vi "_Word Example.vi"() -> ()   [LabVIEW 2017]
uses:
  LabVIEW NPOI/xwpfReader/xwpfReader.lvclass/xwpfReader.ctl
  C:/Users/Neo/Desktop/Dev_Tools_BR/LabVIEW_NPOI/lib/NPOI 2.1.1/NPOI.OOXML.dll
  lib/NPOI 2.1.1/NPOI.OOXML.dll
  LabVIEW NPOI/xwpfReader/Get xwpfRef.vi
  LabVIEW NPOI/Document/Document.lvclass
  LabVIEW NPOI/xwpfReader/xwpfReader.lvclass
panel:
  out "Array 2":i32[][][](array[numeric])
  out "Array 3":string[](array[string])
  out "Array":string[](array[string])
  in  "Text":string="Text ajoute."
  in  "File Path":path
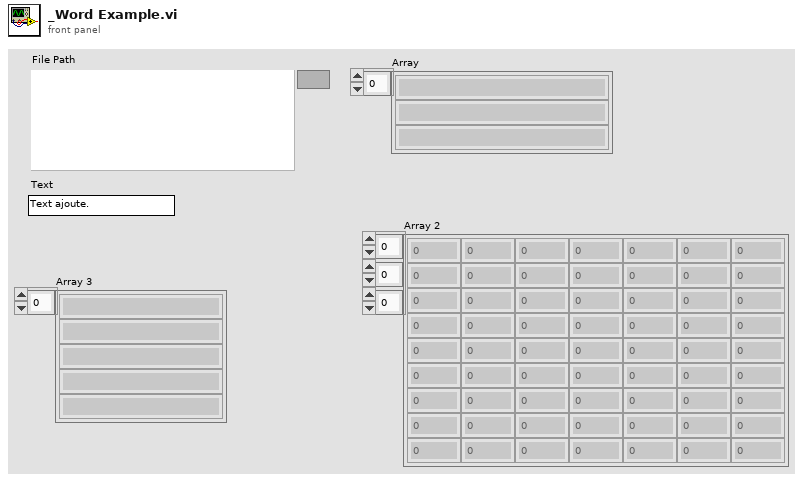
[diagram p1: front panel]
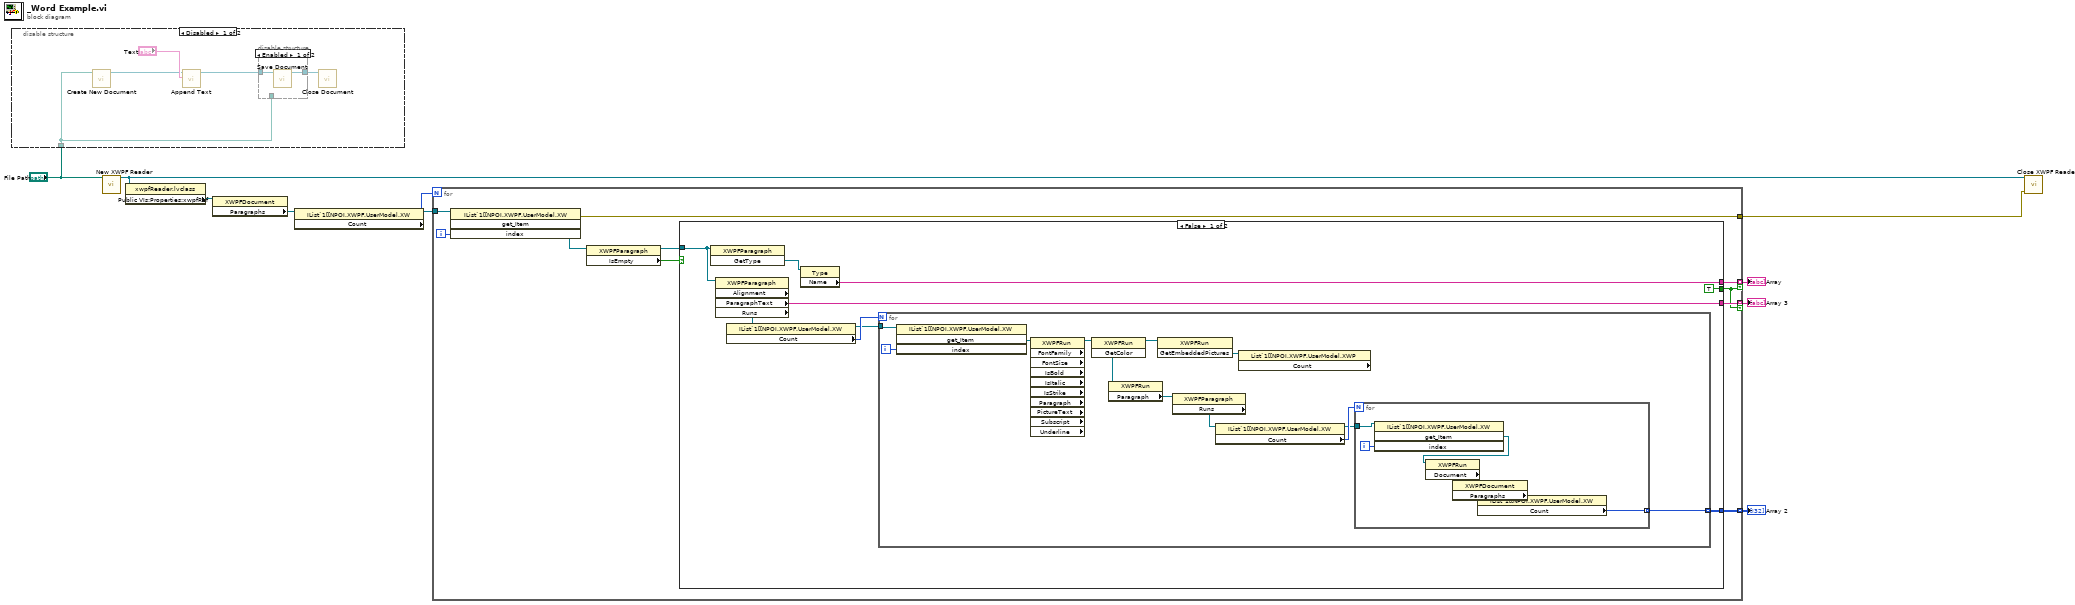
[diagram p0: block diagram]
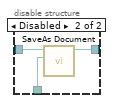
[diagram p3: hidden frame]
diagram:
  n1 = disable-structure shown="Disabled" {
    disable-tunnel: "File Path" -> [w11 _]
    frame Disabled {
      n2 = call "Create New Document.vi"("File Path"=w11) -> ("Document out"=w12:refnum<class "Document.lvclass">)  [unwired: 9 in, 1 out]
      n3 = call "Append Text.vi"("Text"="Text", "Document in"=w12) -> ("Document out"=w14:refnum<class "Document.lvclass">)  [unwired: 8 in, 1 out]
      n4 = disable-structure shown="Enabled" {
        disable-tunnel: [w16 w19] -> w15
        disable-tunnel: w14 -> [w17 w20]
        disable-tunnel: w11 -> [_ w18]
        frame Enabled {
          n5 = call "Save Document.vi"("Document in"=w17) -> ("Document out"=w16:refnum<class "Document.lvclass">)  [unwired: 9 in, 1 out]
        }
        frame Disabled {
          n6 = call "SaveAs Document.vi"("File Path"=w18, "Document in"=w20) -> ("Document out"=w19:refnum<class "Document.lvclass">)  [unwired: 8 in, 1 out]
        }
      }
      n7 = call "Close Document.vi"("Document in"=w15) -> ()  [unwired: 10 in, 1 out]
    }
    frame Enabled {
    }
  }
  n8 = call "New XWPF Reader.vi"("XWPF File Path"="File Path") -> ("xwpfReader out"=w5:refnum<class "xwpfReader.lvclass">)  [unwired: 9 in, 1 out]
  n9 = property class="xwpfReader.lvclass"(reference=w5) -> ("Public VIs:Properties:xwpfRef"=w1:refnum<k24>)  [unwired: 1 in, 2 out]
  n10 = property class="XWPFDocument"(reference=w1) -> ("Paragraphs"=w9:refnum<k24>)  [unwired: 1 in, 2 out]
  n11 = property class="IList`1[[NPOI.XWPF.UserModel.XW"(reference=w9) -> (reference out=w8:refnum<k24>, "Count"=w7:i32)  [unwired: 1 in, 1 out]
  n12 = for {
    N: w7 -> [_]
    tunnel: w8 -> [w30]
    tunnel: [w27] -> w6
    tunnel: [w24] -> w4 mode=indexing if=w22
    tunnel: [w23] -> w3 mode=indexing if=w22
    tunnel: [w21] -> w2 mode=indexing
    i -> [w29]
    n13 = invoke class="IList`1[[NPOI.XWPF.UserModel.XW" method="get_Item"(reference=w30, "index"=w29) -> (error out=w27:errorcluster, "get_Item"=w28:refnum<k24>)  [unwired: 2 in, 2 out]
    n14 = property class="XWPFParagraph"(reference=w28) -> (reference out=w25:refnum<k24>, "IsEmpty"=w26:bool)  [unwired: 1 in, 1 out]
    n15 = case shown="False" w26 {
      tunnel: w25 -> [w36 _]
      tunnel: [w39 _] -> w24
      tunnel: [TRUE _] -> w22
      tunnel: [w35 _] -> w23
      tunnel: [w31 _] -> w21
      frame False {
        n16 = invoke class="XWPFParagraph" method="GetType"(reference=w36) -> ("GetType"=w38:refnum<k24>)  [unwired: 2 in, 2 out]
        n17 = property class="XWPFParagraph" props=["Alignment", "ParagraphText", "Runs"](reference=w36) -> ("ParagraphText"=w35:string, "Runs"=w34:refnum<k24>)  [unwired: 1 in, 3 out]
        n18 = property class="IList`1[[NPOI.XWPF.UserModel.XW"(reference=w34) -> (reference out=w32:refnum<k24>, "Count"=w33:i32)  [unwired: 1 in, 1 out]
        n19 = property class="Type"(reference=w38) -> ("Name"=w39:string)  [unwired: 1 in, 2 out]
        n20 = for {
          N: w33 -> [_]
          tunnel: w32 -> [w51]
          tunnel: [w40] -> w31 mode=indexing
          i -> [w50]
          n21 = invoke class="IList`1[[NPOI.XWPF.UserModel.XW" method="get_Item"(reference=w51, "index"=w50) -> ("get_Item"=w49:refnum<k24>)  [unwired: 2 in, 3 out]
          n22 = property class="XWPFRun" props=["FontFamily", "FontSize", "IsBold", "IsItalic", "IsStrike", "Paragraph", "PictureText", "Subscript", "Underline"](reference=w49) -> (reference out=w48:refnum<k24>)  [unwired: 1 in, 10 out]
          n23 = invoke class="XWPFRun" method="GetColor"(reference=w48) -> (reference out=w47:refnum<k24>)  [unwired: 2 in, 2 out]
          n24 = invoke class="XWPFRun" method="GetEmbeddedPictures"(reference=w47) -> (reference out=w45:refnum<k24>, "GetEmbeddedPictures"=w46:refnum<k24>)  [unwired: 2 in, 1 out]
          n25 = property class="XWPFRun"(reference=w45) -> ("Paragraph"=w44:refnum<k24>)  [unwired: 1 in, 2 out]
          n26 = property class="XWPFParagraph"(reference=w44) -> ("Runs"=w43:refnum<k24>)  [unwired: 1 in, 2 out]
          n27 = property class="IList`1[[NPOI.XWPF.UserModel.XW"(reference=w43) -> (reference out=w41:refnum<k24>, "Count"=w42:i32)  [unwired: 1 in, 1 out]
          n28 = property class="List`1[[NPOI.XWPF.UserModel.XWP" props=["Count"](reference=w46) -> ()  [unwired: 1 in, 3 out]
          n29 = for {
            N: w42 -> [_]
            tunnel: w41 -> [w57]
            tunnel: [w52] -> w40 mode=indexing
            i -> [w56]
            n30 = invoke class="IList`1[[NPOI.XWPF.UserModel.XW" method="get_Item"(reference=w57, "index"=w56) -> ("get_Item"=w55:refnum<k24>)  [unwired: 2 in, 3 out]
            n31 = property class="XWPFRun"(reference=w55) -> ("Document"=w54:refnum<k24>)  [unwired: 1 in, 2 out]
            n32 = property class="XWPFDocument"(reference=w54) -> ("Paragraphs"=w53:refnum<k24>)  [unwired: 1 in, 2 out]
            n33 = property class="IList`1[[NPOI.XWPF.UserModel.XW"(reference=w53) -> ("Count"=w52:i32)  [unwired: 1 in, 2 out]
          }
        }
      }
      frame True {
      }
    }
  }
  "Array" <- w4
  "Array 3" <- w3
  "Array 2" <- w2
  n34 = call "Close XWPF Reader.vi"("error in (no error)"=w6, "xwpfReader in"=w5) -> ()  [unwired: 8 in, 2 out]
